vi "SR_MU-Edit_Op.vi"(10 "Index":i32, 11 "Mission In":T1[](array[typedef]) {"GPS Longitude" format="%.6g"; "GPS Latitude" format="%.6g"}) -> (1 "Add?":bool, 2 "Output":T1 {"GPS Longitude" format="%.6g"; "GPS Latitude" format="%.6g"}, 3 "Mission Out":T1[](array[typedef]) {"GPS Longitude" format="%.6g"; "GPS Latitude" format="%.6g"})   [LabVIEW 2015, in "Shore Library.lvlib"]
uses:
  Shore Library.lvlib
  RDS Mission Controller Actor/MissionOp.ctl
  RDS Mission Controller Actor/RDS Mission Controller Actor.lvlib
panel:
  out "Operation Index":i32
  in  "btn_cancel":bool
  in  "btn_add":bool
  in  "Longitude":dbl
  in  "Latitude":dbl
  in  "Throttle":i16
  in  "Duration (s)":u16
  in  "MissionOp Type":T2(ring)
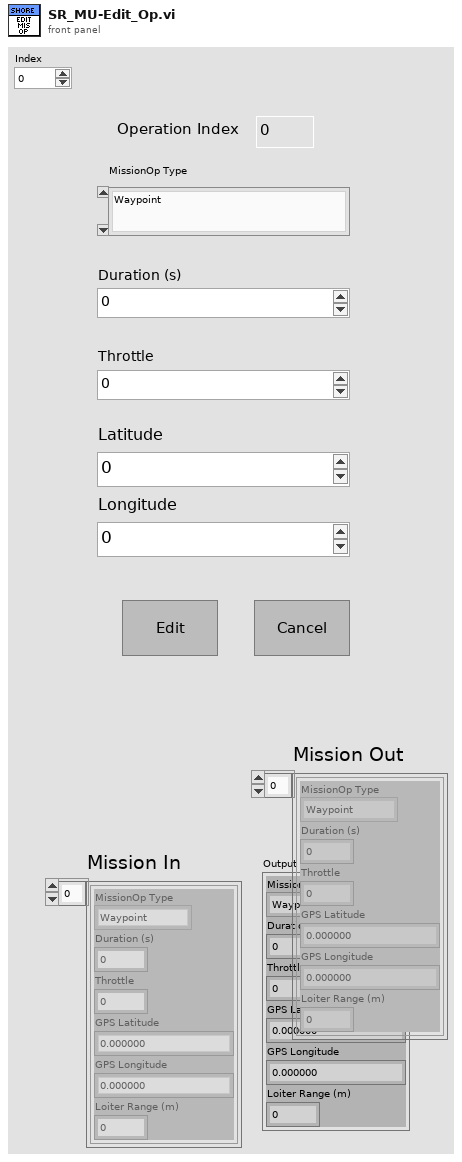
[diagram p1: front panel]
types:
  T1 = typedef "RDS Mission Controller Actor.lvlib/MissionOp.ctl" = cluster{"MissionOp Type":enum16{"Waypoint", "Loiter", "Wait", "Deploy AIP", "Stow AIP"}, "Duration (s)":u16, "Throttle":i16, "GPS Latitude":dbl, "GPS Longitude":dbl, "Loiter Range (m)":u16}
  T2 = enum16{"Waypoint", "Loiter", "Wait", "Deploy AIP", "Stow AIP"}
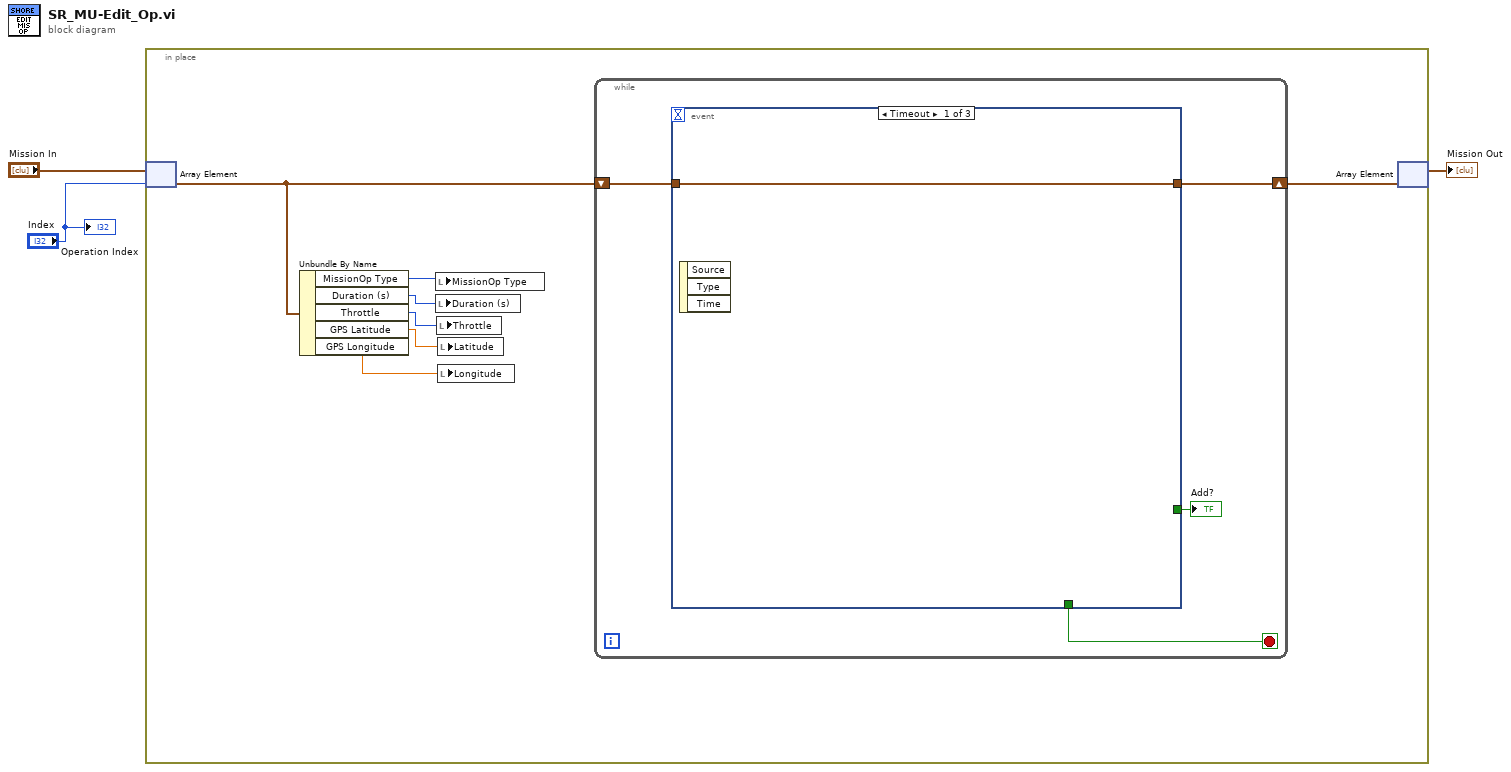
[diagram p0: block diagram]
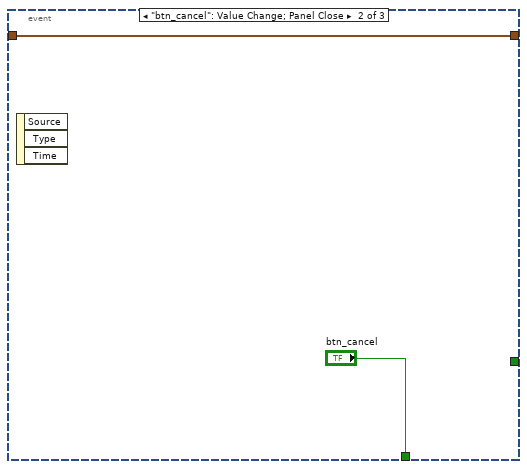
[diagram p2: hidden frame]
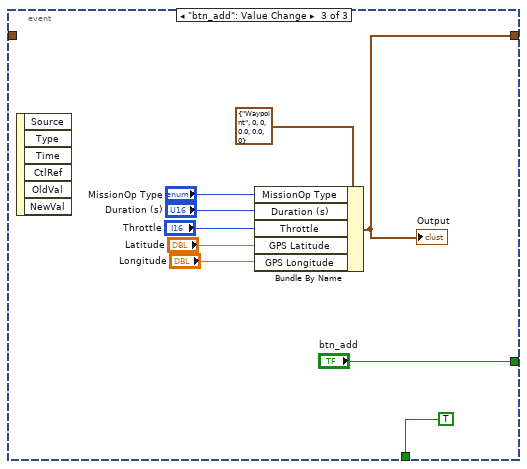
[diagram p3: hidden frame]
diagram:
  n1 = in-place {
    n2 = in-place-array #1("Mission In", "Index") -> (w10:T1)
    n3 = Unbundle By Name(w10) -> ("MissionOp Type"=w8:T2, "Duration (s)"=w7:u16, "Throttle"=w6:i16, "GPS Latitude"=w5:dbl, "GPS Longitude"=w4:dbl)
    n4 = local write "MissionOp Type"(w8) -> ()
    n5 = local write "Duration (s)"(w7) -> ()
    n6 = local write "Throttle"(w6) -> ()
    n7 = local write "Latitude"(w5) -> ()
    n8 = local write "Longitude"(w4) -> ()
    n9 = while {
      shift-right: [w11] -> w9
      shift-left: w10 -> [w12]
      stop <- w14 stop-if-true
      n10 = event shown="[0] Timeout" {
        selector: _ -> [_ _ _]
        dyn-events: _ -> [_ _ _]
        timeout: _ -> [_ _ _]
        tunnel: [_ _ "btn_add"] -> w13
        tunnel: [_ "btn_cancel" TRUE ("btn_add")] -> w14
        tunnel: w12 -> [w15 w16 _]
        tunnel: [w15 w16 w18] -> w11
        event Timeout {
          n11 = event-data() -> ()  [unwired: 1 in, 3 out]
        }
        event "btn_cancel": Value Change; Panel Close {
          n12 = event-data() -> ()  [unwired: 1 in, 3 out]
        }
        event "btn_add": Value Change {
          n13 = event-data() -> ()  [unwired: 1 in, 6 out]
          n14 = Bundle By Name(cluster=T1 {"MissionOp Type"=enum."Waypoint", "Duration (s)"=0, "Throttle"=0, "GPS Latitude"=0.0, "GPS Longitude"=0.0, "Loiter Range (m)"=0} ("MissionOp"), "MissionOp Type"="MissionOp Type", "Duration (s)"="Duration (s)", "Throttle"="Throttle", "GPS Latitude"="Latitude", "GPS Longitude"="Longitude") -> (w18:T1)
          "Output" <- w18
        }
      }
      "Add?" <- w13
    }
    n15 = in-place-array #1(w9) -> (→"Mission Out":T1[])  [unwired: 1 out]
  }
  "Operation Index" <- "Index"
